vi "Set VPP.vi"(8 "error in (no error)":errorcluster, 10 "VPP":dbl, 11 "Generador de funciones in":refnum<class "Generador de funciones.lvclass">) -> (0 "error out":errorcluster, 3 "Generador de funciones out":refnum<class "Generador de funciones.lvclass">)   [LabVIEW 2020, in "Generador de funciones.lvclass"]
uses:
  Generador de funciones.lvclass
  Generador de funciones.lvclass/Generador de funciones.ctl
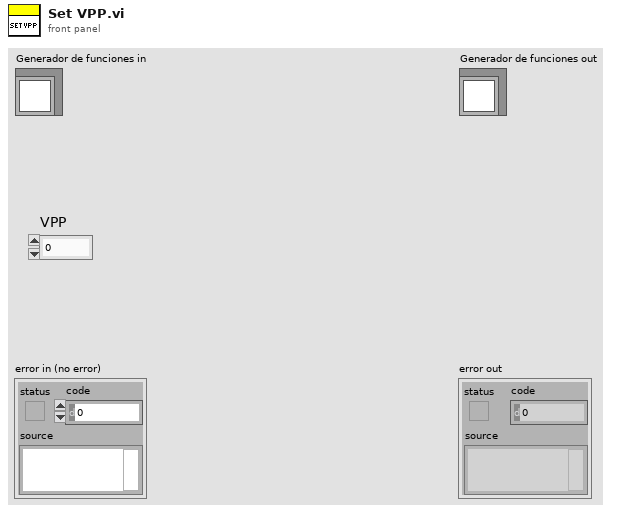
[diagram p1: front panel]
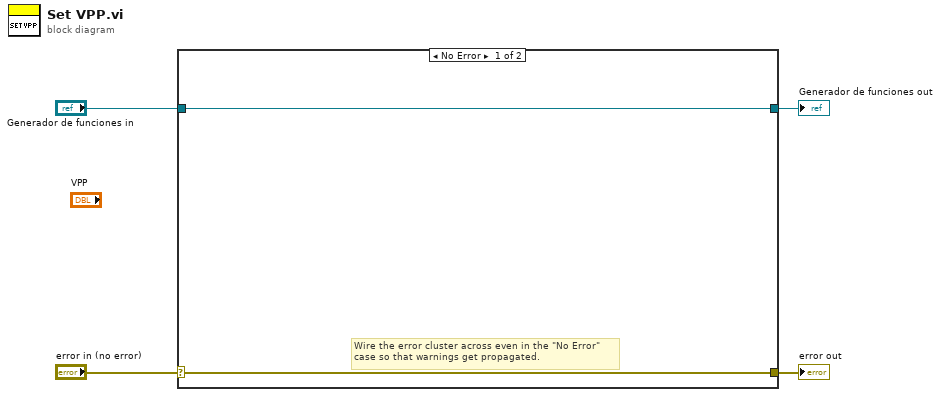
[diagram p0: block diagram]
diagram:
  n1 = case shown="No Error" "error in (no error)" {
    selector: "error in (no error)" -> [w5 w8]
    tunnel: [w5 w8] -> w3
    tunnel: [w6 w7] -> w1
    tunnel: "Generador de funciones in" -> [w6 w7]
    frame No Error {
      # "Wire the error cluster across even in the \"No Error\"\ncase so that warnings get propagated."
    }
    frame Error {
    }
  }
  "error out" <- w3
  "Generador de funciones out" <- w1
